vi "Mutate System Definition File.vi"(8 "error in (no error)":errorcluster, 11 "Original System Definition File":path) -> (0 "error out":errorcluster, 3 "Mutated System Definition File":path)   [LabVIEW 2027, in "Embedded Data Logger Unit Tests.lvclass"]
uses:
  Embedded Data Logger Unit Tests.lvclass
  Embedded Data Logger Unit Tests.lvclass/Embedded Data Logger Unit Tests.ctl
  System Explorer/Embedded Data Logger System Explorer.lvlib
  C:/NetCore/niveristand-embedded-data-logger-custom-device/Source/Tests/Unit/Mutate System Definition File.vi/NationalInstruments.VeriStand.SystemDefinitionAPI
  NationalInstruments.VeriStand.SystemDefinitionAPI
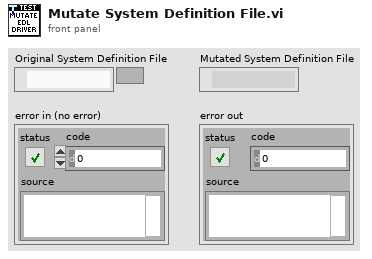
[diagram p1: front panel]
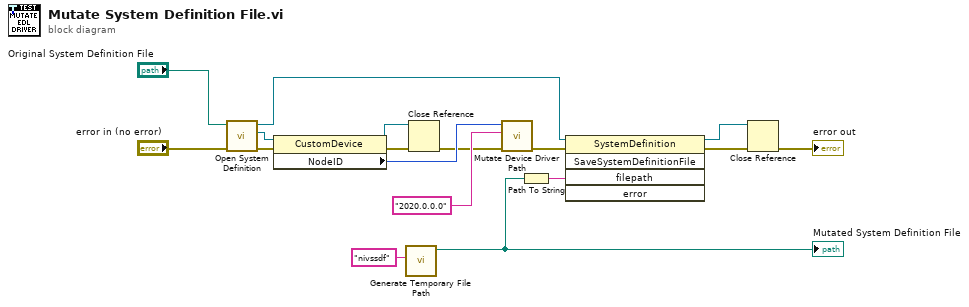
[diagram p0: block diagram]
diagram:
  n1 = call "Open System Definition.vi"("error in (no error)"="error in (no error)", "System Definition File"="Original System Definition File") -> ("error out"=w17:errorcluster, "NationalInstruments.VeriStand.SystemDefinitionAPI.CustomDevice"=w15:refnum<k39>, "NationalInstruments.VeriStand.SystemDefinitionAPI.SystemDefinition"=w8:refnum<k39>)  [unwired: 7 in]
  n2 = property class="CustomDevice"(reference=w15, error in=w17) -> (reference out=w1:refnum<k39>, error out=w3:errorcluster, "NodeID"=w16:u64)
  n3 = call <vilib>:"Generate Temporary File Path.vi"("Temporary File Extension (tmp)"="nivssdf") -> ("Unique Temporary File Path"=w13:path)  [unwired: 9 in, 1 out]
  "Mutated System Definition File" <- w13
  n4 = Close Reference(reference=w1, error in (no error)=w3) -> (error out=w2:errorcluster)
  n5 = call "Mutate Device Driver Path.vi"("error in (no error)"=w2, "Version"="2020.0.0.0", "Device Ref in"=w16) -> ("error out"=w10:errorcluster)  [unwired: 7 in, 1 out]
  n6 = Path To String(path=w13) -> (string=w12:string)
  n7 = invoke class="SystemDefinition" method="SaveSystemDefinitionFile"(reference=w8, error in=w10, "filepath"=w12) -> (reference out=w9:refnum<k39>, error out=w11:errorcluster)  [unwired: 2 in, 3 out]
  n8 = Close Reference(reference=w9, error in (no error)=w11) -> (error out=→"error out":errorcluster)
